vi "Convert Keyboard Event Data.vi"(11 "Event Data":u8[](array[numeric]) format="%.0x") -> (3 "Keyboard Event":T1 {"Padding 2" format="%.0x"; "Padding 1" format="%.0x"; "Window ID" format="%.0x"; "Type" format="%.0x"; "Key Sym"."Unused" format="%.0x"; "Key Sym"."Mod" format="%.0x"; "Key Sym"."Sym" format="%.0x"; "Key Sym"."Scan Code" format="%.0x"})   [LabVIEW 2015, in "LibSDL2.lvlib"]
uses:
  LibSDL2.lvlib
  Controls/Keyboard Event.ctl
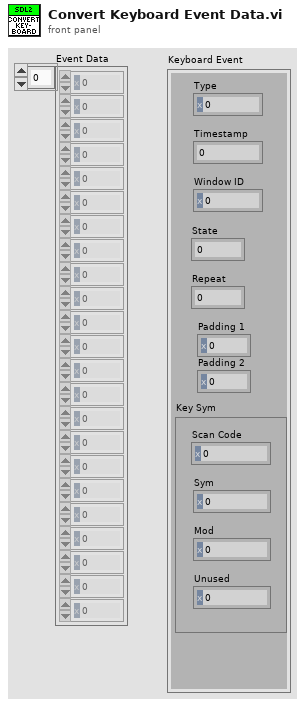
[diagram p1: front panel]
types:
  T1 = typedef "LibSDL2.lvlib/Keyboard Event.ctl" = cluster{"Type":u32, "Timestamp":u32, "Window ID":u32, "State":u8, "Repeat":u8, "Padding 1":u8, "Padding 2":u8, "Key Sym":cluster{"Scan Code":u32, "Sym":i32, "Mod":u16, "Unused":u32}}
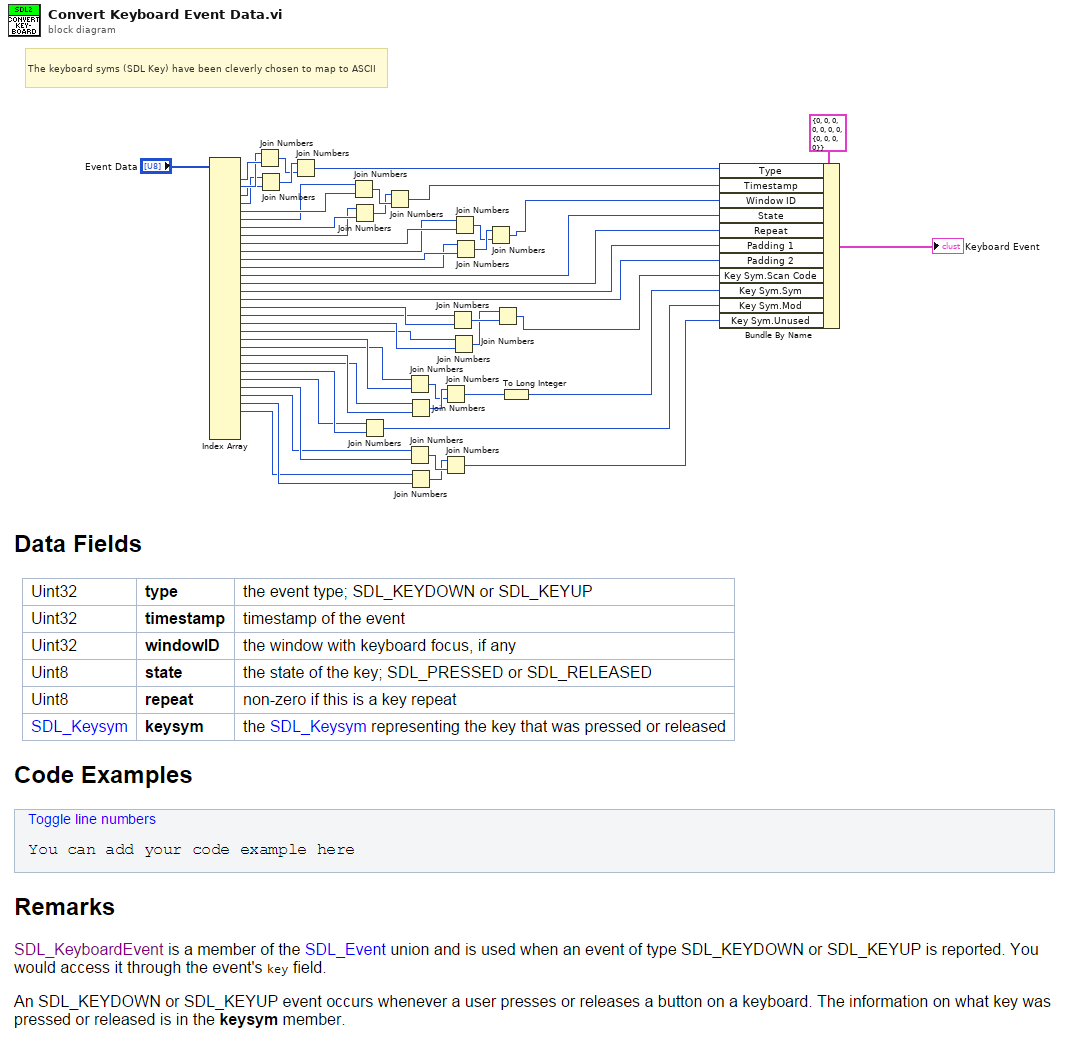
[diagram p0: block diagram]
diagram:
  # "The keyboard syms (SDL Key) have been cleverly chosen to map to ASCII"
  n1 = Index Array(array="Event Data") -> (element #1=w50:u8, element #2=w49:u8, element #3=w47:u8, element #4=w48:u8, element #5=w41:u8, element #6=w40:u8, element #7=w39:u8, element #8=w38:u8, element #9=w34:u8, element #10=w33:u8, element #11=w32:u8, element #12=w31:u8, element #13=w29:u8, element #14=w28:u8, element #15=w22:u8, element #16=w21:u8, element #17=w20:u8, element #18=w19:u8, element #19=w18:u8, element #20=w17:u8, element #21=w13:u8, element #22=w12:u8, element #23=w11:u8, element #24=w10:u8, element #25=w9:u8, element #26=w8:u8, element #27=w5:u8, element #28=w4:u8, element #29=w3:u8, element #30=w2:u8)  [unwired: 33 in, 3 out]
  n2 = Join Numbers(hi=w49, lo=w50) -> ((hi.lo)=w45:u16)
  n3 = Join Numbers(hi=w48, lo=w47) -> ((hi.lo)=w46:u16)
  n4 = Join Numbers(hi=w46, lo=w45) -> ((hi.lo)=w44:u32)
  n5 = Join Numbers(hi=w40, lo=w41) -> ((hi.lo)=w43:u16)
  n6 = Join Numbers(hi=w38, lo=w39) -> ((hi.lo)=w42:u16)
  n7 = Join Numbers(hi=w8, lo=w9) -> ((hi.lo)=w23:u16)
  n8 = Join Numbers(hi=w42, lo=w43) -> ((hi.lo)=w37:u32)
  n9 = Join Numbers(hi=w12, lo=w13) -> ((hi.lo)=w26:u16)
  n10 = Join Numbers(hi=w4, lo=w5) -> ((hi.lo)=w7:u16)
  n11 = Join Numbers(hi=w10, lo=w11) -> ((hi.lo)=w27:u16)
  n12 = Join Numbers(hi=w2, lo=w3) -> ((hi.lo)=w6:u16)
  n13 = Join Numbers(hi=w27, lo=w26) -> ((hi.lo)=w25:u32)
  n14 = Join Numbers(hi=w6, lo=w7) -> ((hi.lo)=w1:u32)
  n15 = Join Numbers(hi=w19, lo=w20) -> ((hi.lo)=w16:u16)
  n16 = Join Numbers(hi=w17, lo=w18) -> ((hi.lo)=w15:u16)
  n17 = Join Numbers(hi=w33, lo=w34) -> ((hi.lo)=w35:u16)
  n18 = Join Numbers(hi=w31, lo=w32) -> ((hi.lo)=w36:u16)
  n19 = Join Numbers(hi=w36, lo=w35) -> ((hi.lo)=w30:u32)
  n20 = Join Numbers(hi=w15, lo=w16) -> ((hi.lo)=w14:u32)
  n21 = To Long Integer(number=w25) -> (32bit integer=w24:i32)
  n22 = Bundle By Name(cluster=T1 {"Type"=0, "Timestamp"=0, "Window ID"=0, "State"=0, "Repeat"=0, "Padding 1"=0, "Padding 2"=0, "Key Sym"={"Scan Code"=0, "Sym"=0, "Mod"=0, "Unused"=0}} ("Keyboard Event"), "Type"=w44, "Timestamp"=w37, "Window ID"=w30, "State"=w29, "Repeat"=w28, "Padding 1"=w22, "Padding 2"=w21, "Key Sym.Scan Code"=w14, "Key Sym.Sym"=w24, "Key Sym.Mod"=w23, "Key Sym.Unused"=w1) -> (→"Keyboard Event":T1)
